vi "Left_to_Negative_Left.vi"(2 "negative left in":dbl, 3 "positive left in":dbl) -> (0 "positive left out":dbl, 1 "negative left out":dbl)   [LabVIEW 2009]
uses:
  <vilib>/gmath/NI_Gmath.lvlib
panel:
  in  "Left / Negative Left Correlation":cluster{"negative left":dbl, "left":dbl}[](array[cluster])=[{"negative left"=2.5, "left"=2.5}, {"negative left"=2.39, "left"=2.75}, {"negative left"=2.12, "left"=3.0}, {"negative left"=1.89, "left"=3.25}, {"negative left"=1.65, "left"=3.5}, {"negative left"=1.4, "left"=3.75}, {"negative left"=1.16, "left"=4.0}, {"negative left"=0.92, "left"=4.25}, {"negative left"=0.66, "left"=4.5}, {"negative left"=0.58, "left"=4.75}, {"negative left"=0.57, "left"=5.0}]
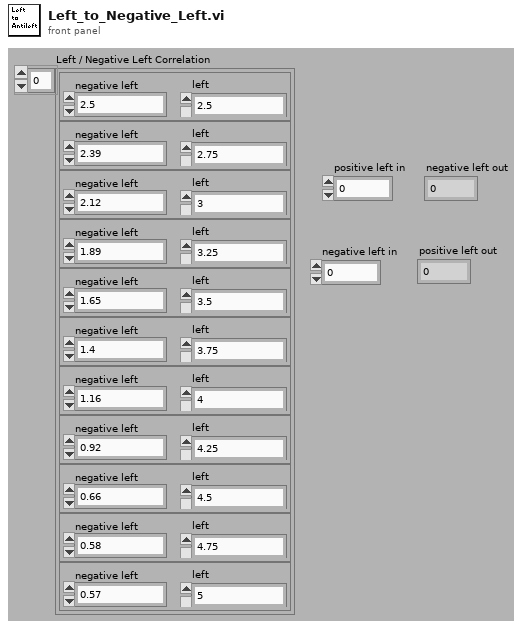
[diagram p1: front panel]
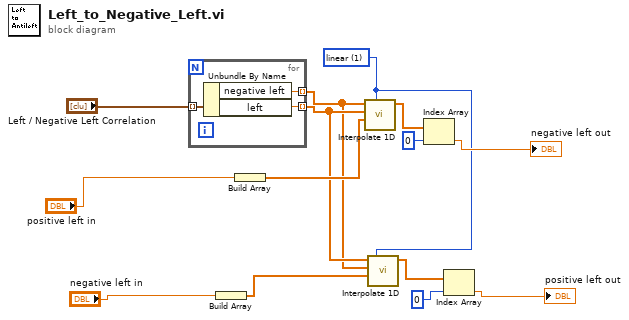
[diagram p0: block diagram]
diagram:
  w7 = 1 items=["nearest", "linear", "spline", "cubic Hermite", "Lagrange"] ("method")
  n1 = for {
    tunnel: "Left / Negative Left Correlation" -> [w17] mode=indexing
    tunnel: [w16] -> w5 mode=indexing
    tunnel: [w15] -> w6 mode=indexing
    n2 = Unbundle By Name(w17) -> ("negative left"=w16:dbl, "left"=w15:dbl)
  }
  n3 = Build Array("negative left in") -> (w4:dbl[])
  n4 = Build Array("positive left in") -> (w9:dbl[])
  n5 = call <vilib>:"Interpolate 1D.vi"("method"=w7, "xi"=w9, "X"=w6, "Y"=w5) -> ("yi"=w13:dbl[])  [unwired: 5 in, 2 out]
  n6 = call <vilib>:"Interpolate 1D.vi"("method"=w7, "xi"=w4, "X"=w5, "Y"=w6) -> ("yi"=w2:dbl[])  [unwired: 5 in, 2 out]
  n7 = Index Array(array=w13, index=0) -> (element=→"negative left out":dbl)
  n8 = Index Array(array=w2, index=0) -> (element=→"positive left out":dbl)
